vi "ManualThresholdLocalization-3.vi"(4 "[IN] Gauss Filter":bool, 5 "[IN] Settings":T1={"Objects"=0, "Threshold"=128, "Reject Border"=FALSE, "Fill Holes"=FALSE, "Min Object Size"=FALSE, "Min Size"=3, "Max Object Size"=FALSE, "Max Size"=100, "Show Search Area"=FALSE, "Show Center"=TRUE, "Show Bounding Box"=TRUE} {"Objects" items=["Bright Objects", "Dark Objects"]; "Threshold" min=1 max=999999999 step=1; "Max Size" min=1 max=999999999 step=1; "Min Size" min=1 max=999999999 step=1}, 6 "[IN] Autothreshold Images \nInstead Of Generated U8":bool, 7 "[IN] Median Filter":bool, 8 "error IN":errorcluster, 10 "[IN] Binarized Image":T2, 11 "[IN] Source Image":T2) -> (0 "error OUT":errorcluster, 2 "[OUT] X,Y Coordinates":dbl[](array[numeric]))   [LabVIEW 2020]
uses:
  <vilib>/vision/Image Controls.llb/IMAQ Image.ctl
  <vilib>/vision/Image Controls.llb/IMAQ Rounding Mode.ctl
  <vilib>/vision/NI_Vision_Development_Module.lvlib
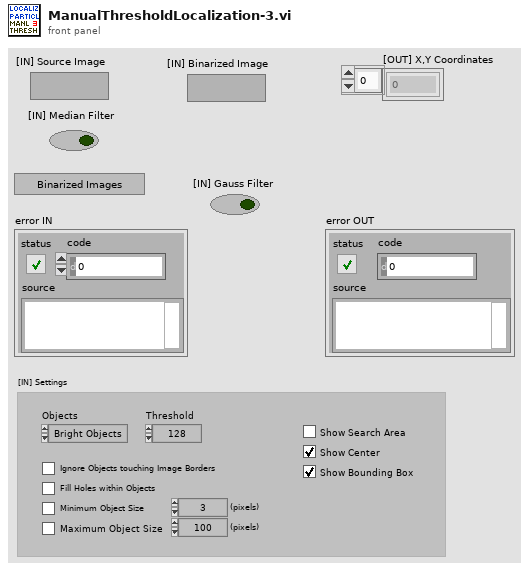
[diagram p1: front panel]
types:
  T1 = cluster{"Objects":u16, "Threshold":i32, "Reject Border":bool, "Fill Holes":bool, "Min Object Size":bool, "Min Size":i32, "Max Object Size":bool, "Max Size":i32, "Show Search Area":bool, "Show Center":bool, "Show Bounding Box":bool}
  T2 = typedef "IMAQ Image.ctl" = refnum<image>
  T3 = typedef "Image Type" = u32
  T4 = cluster{"X Size":i32, "Y Size":i32, "Order #":i32}
  T5 = typedef "IMAQ Rounding Mode.ctl" = enum16{"Optimize", "Truncate"}
  T6 = cluster{"Object Center":cluster{"X":sgl, "Y":sgl}, "Bounding Box":cluster{"X Left":i32, "Y Top":i32, "X Right":i32, "Y Bottom":i32}, "Area":sgl, "Orientation":sgl, "Aspect Ratio":sgl, "Nb Holes":i32}[]
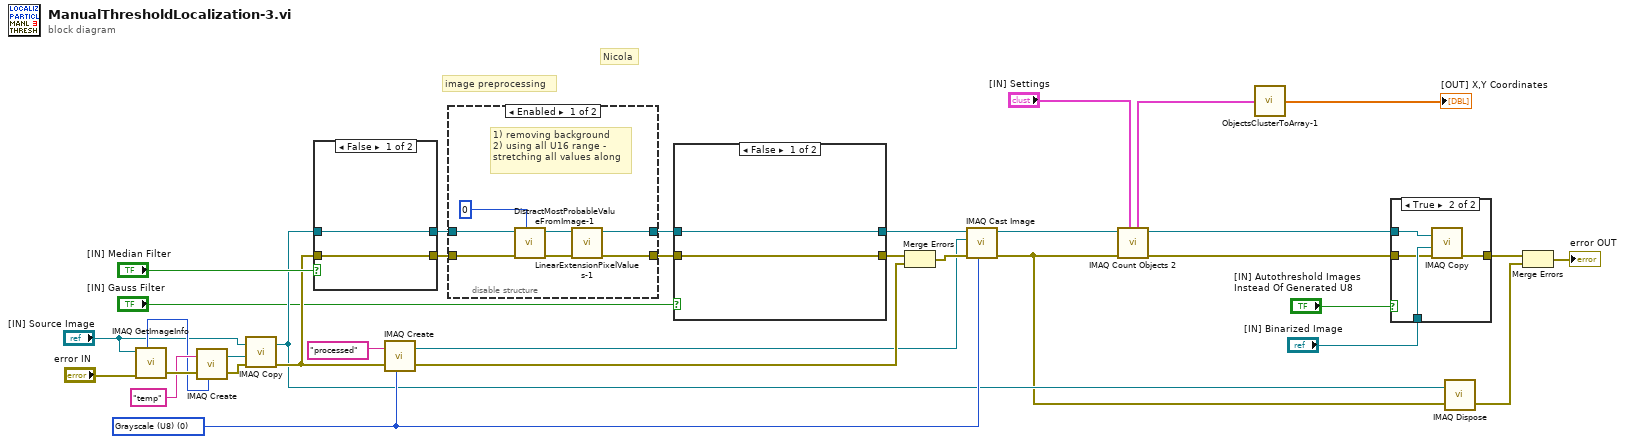
[diagram p0: block diagram]
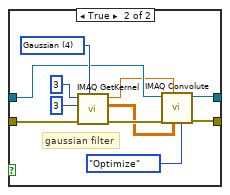
[diagram p3: hidden frame]
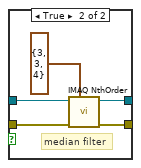
[diagram p4: hidden frame]
diagram:
  w30 = T3 0 items=["Grayscale (U8)", "Grayscale (I16)", "Grayscale (SGL)", "Complex (CSG)", "RGB (U32)", "HSL (U32)", "RGB (U64)", "Grayscale (U16)"] ("Image Type")
  # "Nicola"
  # "image preprocessing"
  n1 = call "IMAQ GetImageInfo"("error in (no error)"="error IN", "Image"="[IN] Source Image") -> ("error out"=w26:errorcluster, "Image Type"=w24:T3)  [unwired: 2 in, 6 out]
  n2 = call "IMAQ Create"("Image Name"="temp", "Image Type"=w24, "error in (no error)"=w26) -> ("New Image"=w22:T2, "error out"=w23:errorcluster)  [unwired: 2 in]
  n3 = call "IMAQ Copy"("error in (no error)"=w23, "Image Dst"=w22, "Image Src"="[IN] Source Image") -> ("error out"=w20:errorcluster, "Image Dst Out"=w19:T2)  [unwired: 3 in]
  n4 = case shown="False" "[IN] Median Filter" {
    tunnel: w19 -> [w36 w40]
    tunnel: w20 -> [w35 w39]
    tunnel: [w36 w38] -> w14
    tunnel: [w35 w37] -> w13
    frame False {
    }
    frame True {
      # "median filter"
      n5 = call "IMAQ NthOrder"("Image Src"=w40, "Size & Order #"=T4 {"X Size"=3, "Y Size"=3, "Order #"=4}, "error in (no error)"=w39) -> ("Image Dst Out"=w38:T2, "error out"=w37:errorcluster)  [unwired: 4 in]
    }
  }
  n6 = call "IMAQ Create"("Image Name"="processed", "Image Type"=w30, "error in (no error)"=w20) -> ("New Image"=w15:T2, "error out"=w29:errorcluster)  [unwired: 2 in]
  n7 = disable-structure shown="Enabled" {
    disable-tunnel: w14 -> [w47 w50]
    disable-tunnel: w13 -> [w46 w49]
    disable-tunnel: [w45 w50] -> w12
    disable-tunnel: [w44 w49] -> w11
    frame Enabled {
      # "1) removing background\n2) using all U16 range - \nstretching all values along"
      n8 = call "DistractMostProbableValueFromImage-1.vi"("[IN] # Iteration"=0, "error in"=w46, "[IN] Max Projected Image"=w47) -> ("error out"=w42:errorcluster, "[OUT] Processed Image"=w43:T2)  [unwired: 6 in, 1 out]
      n9 = call "LinearExtensionPixelValues-1.vi"("error in"=w42, "[IN] Max Projected Image"=w43) -> ("error out"=w44:errorcluster, "[OUT] Processed Image"=w45:T2)  [unwired: 8 in]
    }
    frame Disabled {
    }
  }
  n10 = case shown="False" "[IN] Gauss Filter" {
    tunnel: w12 -> [w52 w58]
    tunnel: w11 -> [w51 w60]
    tunnel: [w52 w55] -> w10
    tunnel: [w51 w54] -> w9
    frame False {
    }
    frame True {
      w61 = u16 4 items=["Gradient"=1, "Laplacian"=2, "Smoothing"=3, "Gaussian"=4] ("Kernel Family")
      # "gaussian filter"
      n11 = call "IMAQ GetKernel"("Kernel Family"=w61, "error in (no error)"=w60, "Kernel Number"=3, "Kernel Size (3,5,...)"=3) -> ("error out"=w59:errorcluster, "Kernel"=w56:sgl[][], "Divider"=w57:sgl)  [unwired: 4 in, 1 out]
      n12 = call "IMAQ Convolute"("Rounding Mode"=IMAQ_Rounding_Mode."Optimize", "Kernel"=w56, "Divider (kernel sum)"=w57, "error in (no error)"=w59, "Image Src"=w58) -> ("error out"=w54:errorcluster, "Image Dst Out"=w55:T2)  [unwired: 5 in]
    }
  }
  n13 = Merge Errors(w9, w29) -> (w28:errorcluster)
  n14 = call "IMAQ Cast Image"("Image Type"=w30, "error in (no error)"=w28, "Image Dst"=w15, "Image Src"=w10) -> ("error out"=w2:errorcluster, "Image Dst Out"=w7:T2)  [unwired: 6 in]
  n15 = call "IMAQ Count Objects 2"("Settings"="[IN] Settings", "error in (no error)"=w2, "Image"=w7) -> ("error out"=w4:errorcluster, "Image Out"=w3:T2, "Objects"=w6:T6)  [unwired: 4 in, 2 out]
  n16 = call "ObjectsClusterToArray-1.vi"("[IN] Objects"=w6) -> ("[OUT] X,Y Coordinates"=→"[OUT] X,Y Coordinates":dbl[])
  n17 = case shown="True" "[IN] Autothreshold Images \nInstead Of Generated U8" {
    tunnel: w4 -> [w64 w66]
    tunnel: [w64 w68] -> w17
    tunnel: w3 -> [_ w65]
    tunnel: "[IN] Binarized Image" -> [_ w67]
    frame False {
    }
    frame True {
      n18 = call "IMAQ Copy"("error in (no error)"=w66, "Image Dst"=w67, "Image Src"=w65) -> ("error out"=w68:errorcluster)  [unwired: 3 in, 1 out]
    }
  }
  n19 = call "IMAQ Dispose"("Image"=w19, "error in (no error)"=w2) -> ("error out"=w18:errorcluster)  [unwired: 4 in]
  n20 = Merge Errors(w17, w18) -> (→"error OUT":errorcluster)
